vi "close_connection.vi"(8 "error in (no error)":errorcluster, 11 "TCP Connection in":refnum<class "TCP Connection.lvclass">) -> (0 "error out":errorcluster)   [LabVIEW 2019, in "TCP Connection.lvclass"]
uses:
  TCP Connection.lvclass
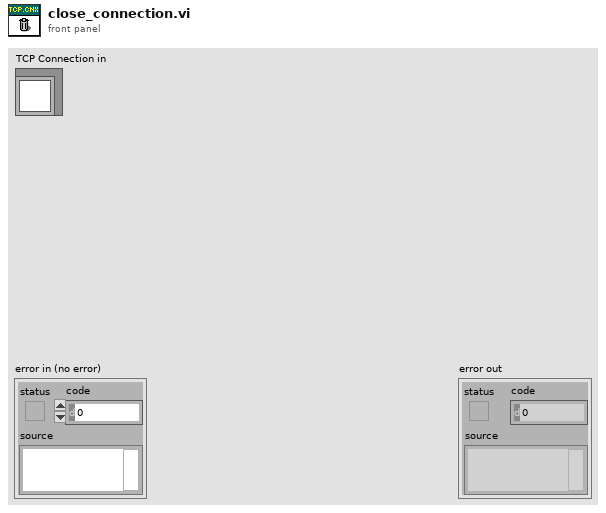
[diagram p1: front panel]
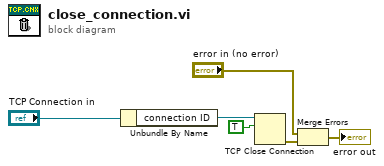
[diagram p0: block diagram]
diagram:
  n1 = Unbundle By Name("TCP Connection in") -> ("connection ID"=w5:refnum<k5>)
  n2 = TCP Close Connection(connection ID=w5, abort (F)=TRUE) -> (error out=w2:errorcluster)  [unwired: 1 in, 1 out]
  n3 = Merge Errors("error in (no error)", w2) -> (→"error out":errorcluster)
